vi "onConnection.vi"(8 "error in (no error)":errorcluster, 11 "Connection.Collection":refnum<class "Connection.Collection.lvclass">) -> (0 "error out":errorcluster, 3 "Connection.Collection":refnum<class "Connection.Collection.lvclass">)   [LabVIEW 2013, in "Connection_GOSPL.lvlib" / "Connection.Collection.lvclass"]
uses:
  Connection.Collection.lvclass
  Connection.Collection.lvclass/Connection.Collection.ctl
  Connection/Connection.lvclass
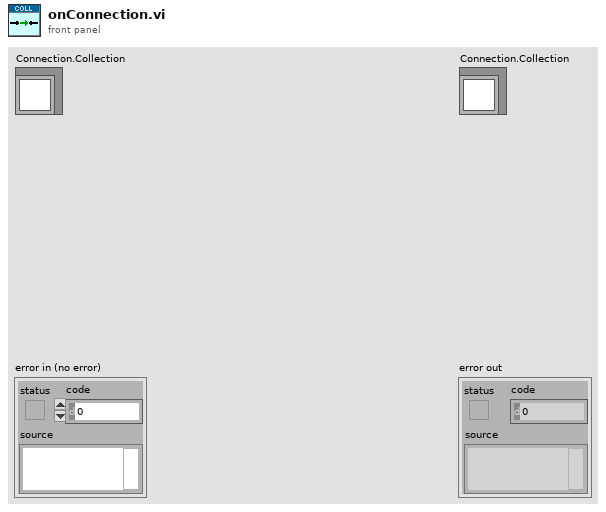
[diagram p1: front panel]
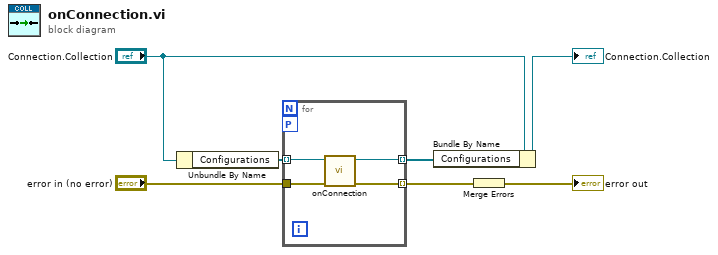
[diagram p0: block diagram]
diagram:
  n1 = Unbundle By Name("Connection.Collection") -> ("Configurations"=w6:refnum<class "Connection.lvclass">[])
  n2 = for {
    tunnel: "error in (no error)" -> [w10]
    tunnel: [w8] -> w2 mode=indexing
    tunnel: [w9] -> w5 mode=indexing
    tunnel: w6 -> [w11] mode=indexing
    workers-P: _ -> [_]
    n3 = call-dynamic "onConnection.vi"("error in (no error)"=w10, "Connection in"=w11) -> ("error out"=w8:errorcluster, "Connection out"=w9:refnum<class "Connection.lvclass">)  [unwired: 8 in]
  }
  n4 = Bundle By Name(cluster="Connection.Collection", "Configurations"=w5) -> (→"Connection.Collection":refnum<class "Connection.Collection.lvclass">)
  n5 = Merge Errors(w2) -> (→"error out":errorcluster)
